vi "CalcCheckboxesFromTree.vi"(8 "error in (no error)":errorcluster, 11 "Tree Reference":refnum<vi>) -> (0 "error out":errorcluster, 1 "Element Status Conditions":T1(array[ring]), 2 "Element Values":enum8{"False", "True", "Mixed"}[](array[ring]))   [LabVIEW 2016, in "CS++MessageMakerMain.lvlib" / "CS++MessageMakerMain.lvclass"]
uses:
  CS++MessageMakerMain.lvclass
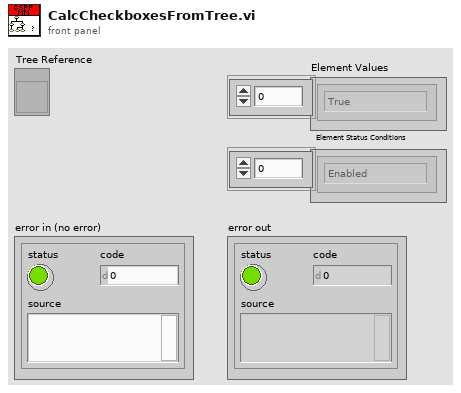
[diagram p1: front panel]
types:
  T1 = enum8{"Enabled", "Disabled", "Disabled and Grayed Out"}[]
  T2 = enum8{"Enabled", "Disabled", "Disabled and Grayed Out"}
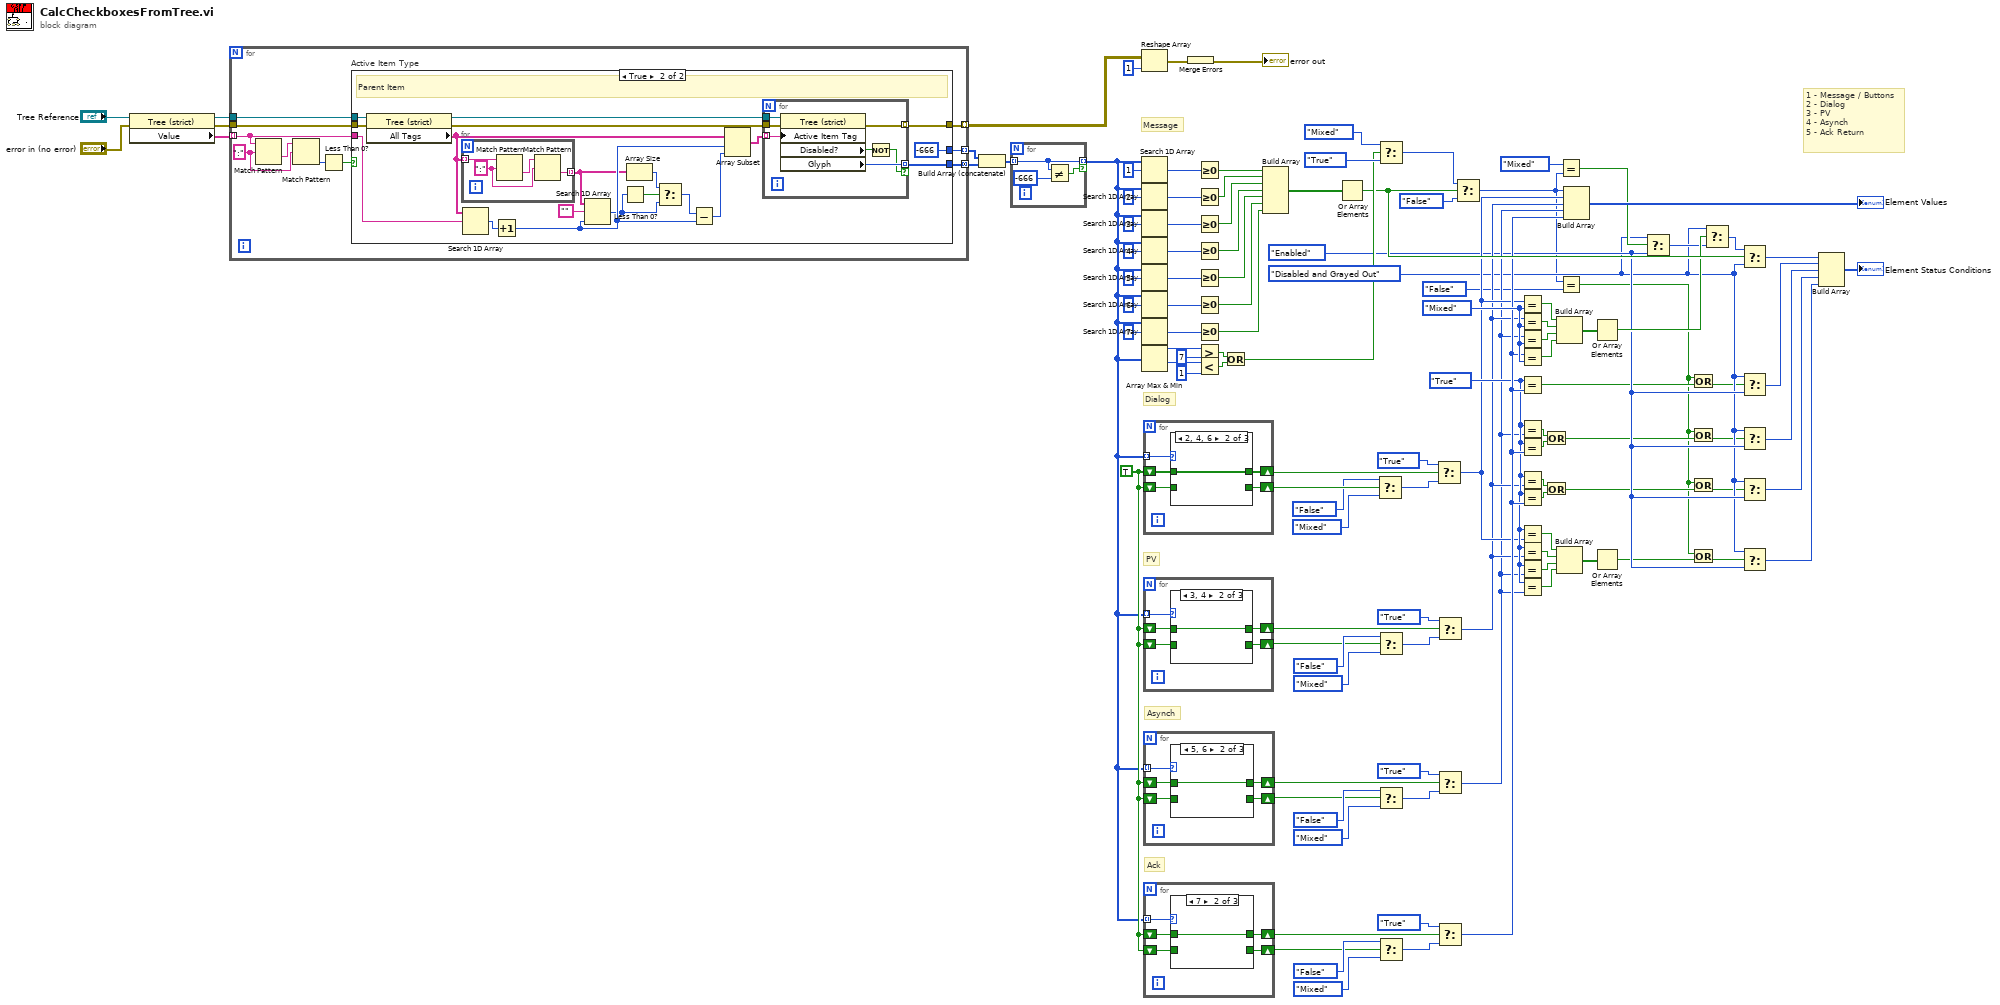
[diagram p0: block diagram]
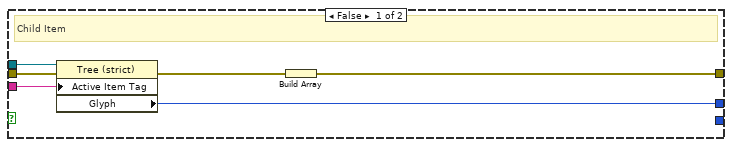
[diagram p2: hidden frame]
diagram:
  w24 = enum8{"False", "True", "Mixed"}."True" ("Element Value")
  w45 = enum8{"False", "True", "Mixed"}."Mixed" ("Element Value")
  w18 = T2."Enabled" ("Element Condition")
  w53 = TRUE
  w16 = T2."Disabled and Grayed Out" ("Element Condition")
  # "Message"
  # "Ack"
  # "Asynch"
  # "PV"
  # "Dialog"
  # "1 - Message / Buttons\n2 - Dialog\n3 - PV\n4 - Asynch\n5 - Ack Return"
  n1 = property class="Tree (strict)"(reference="Tree Reference", error in="error in (no error)") -> (reference out=w113:refnum<vi>, error out=w115:errorcluster, "Value"=w114:string[])
  n2 = for {
    tunnel: w114 -> [w123] mode=indexing
    tunnel: w113 -> [w121]
    tunnel: [w119] -> w15 mode=indexing
    tunnel: [w118] -> w14 mode=concatenating
    tunnel: w115 -> [w122]
    tunnel: [w120] -> w110 mode=indexing
    w126 = ":" ("regular expression")
    n3 = Match Pattern(string=w123, regular expression=w126) -> (after substring=w127:string)  [unwired: 1 in, 3 out]
    n4 = Match Pattern(string=w127, regular expression=w126) -> (offset past match=w125:i32)  [unwired: 1 in, 3 out]
    n5 = Less Than 0?(x=w125) -> (x < 0?=w124:bool)
    n6 = case "Active Item Type" shown="True" w124 {
      tunnel: w121 -> [w132 w152]
      tunnel: w123 -> [w129 w150]
      tunnel: w122 -> [w131 w151]
      tunnel: [w133 w141] -> w120
      tunnel: [_ w140] -> w118
      tunnel: [w128 -666 ("Glyph")] -> w119
      frame False {
        # "Child Item"
        n7 = property class="Tree (strict)"(reference=w132, error in=w131, "Active Item Tag"=w129) -> (error out=w130:errorcluster, "Glyph"=w128:i32)  [unwired: 1 out]
        n8 = Build Array(w130) -> (w133:errorcluster[])
      }
      frame True {
        # "Parent Item"
        n9 = property class="Tree (strict)"(reference=w152, error in=w151) -> (reference out=w144:refnum<vi>, error out=w143:errorcluster, "All Tags"=w147:string[])
        n10 = for {
          tunnel: w147 -> [w154] mode=indexing
          tunnel: [w153] -> w135 mode=indexing
          w155 = ":" ("regular expression")
          n11 = Match Pattern(string=w154, regular expression=w155) -> (after substring=w156:string)  [unwired: 1 in, 3 out]
          n12 = Match Pattern(string=w156, regular expression=w155) -> (after substring=w153:string)  [unwired: 1 in, 3 out]
        }
        n13 = Search 1D Array(1D array=w147, element=w150) -> (index of element=w149:i32)  [unwired: 1 in]
        n14 = Increment(x=w149) -> (x+1=w142:i32)
        n15 = Search 1D Array(1D array=w135, element="", start index (0)=w142) -> (index of element=w138:i32)
        n16 = Less Than 0?(x=w138) -> (x < 0?=w139:bool)
        n17 = Array Size(array=w135) -> (size(s)=w136:i32)
        n18 = Select(t=w136, s=w139, f=w138) -> (s? t:f=w137:i32)
        n19 = Subtract(x=w137, y=w142) -> (x-y=w146:i32)
        n20 = Array Subset(array=w147, index=w142, length=w146) -> (w145:string[])
        n21 = for {
          tunnel: w145 -> [w158] mode=indexing
          tunnel: w144 -> [w163]
          tunnel: w143 -> [w162]
          tunnel: [w160] -> w141 mode=indexing
          tunnel: [w159] -> w140 mode=indexing if=w157
          n22 = property class="Tree (strict)"(reference=w163, error in=w162, "Active Item Tag"=w158) -> (error out=w160:errorcluster, "Disabled?"=w161:bool, "Glyph"=w159:i32)  [unwired: 1 out]
          n23 = Not(x=w161) -> (.not. x?=w157:bool)
        }
      }
    }
  }
  n24 = Build Array (concatenate)(w15, w14) -> (w13:i32[])
  n25 = for {
    tunnel: w13 -> [w165] mode=indexing
    tunnel: [w165] -> w12 mode=indexing if=w164
    n26 = Not Equal?(x=w165, y=-666) -> (x != y?=w164:bool)
  }
  n27 = Reshape Array(w110, 1 ("dimension size")) -> (w111:errorcluster[])
  n28 = Search 1D Array(1D array=w12, element=1) -> (index of element=w101:i32)  [unwired: 1 in]
  n29 = Search 1D Array(1D array=w12, element=2) -> (index of element=w100:i32)  [unwired: 1 in]
  n30 = Search 1D Array(1D array=w12, element=3) -> (index of element=w99:i32)  [unwired: 1 in]
  n31 = Search 1D Array(1D array=w12, element=4) -> (index of element=w98:i32)  [unwired: 1 in]
  n32 = Search 1D Array(1D array=w12, element=5) -> (index of element=w97:i32)  [unwired: 1 in]
  n33 = Search 1D Array(1D array=w12, element=6) -> (index of element=w96:i32)  [unwired: 1 in]
  n34 = Search 1D Array(1D array=w12, element=7) -> (index of element=w95:i32)  [unwired: 1 in]
  n35 = Array Max & Min(array=w12) -> (max value=w81:i32, min value=w80:i32)  [unwired: 2 out]
  n36 = for {
    tunnel: w12 -> [w171] mode=indexing
    shift-right: [w169] -> w71
    shift-left: w53 -> [w170]
    shift-right: [w167] -> w68
    shift-left: w53 -> [w168]
    n37 = case shown="2, 4, 6" w171 {
      tunnel: w170 -> [w172 w174 _]
      tunnel: [w172 w174 _] -> w169
      tunnel: w168 -> [w173 _ w175]
      tunnel: [w173 _ w175] -> w167
      frame Default {
      }
      frame 2, 4, 6 {
      }
      frame 0, 1, 3, 5, 7 {
      }
    }
  }
  n38 = for {
    tunnel: w12 -> [w180] mode=indexing
    shift-right: [w178] -> w61
    shift-left: w53 -> [w179]
    shift-right: [w176] -> w60
    shift-left: w53 -> [w177]
    n39 = case shown="3, 4" w180 {
      tunnel: w179 -> [w181 w183 _]
      tunnel: [w181 w183 _] -> w178
      tunnel: w177 -> [w182 _ w184]
      tunnel: [w182 _ w184] -> w176
      frame Default {
      }
      frame 3, 4 {
      }
      frame 0..2, 5..7 {
      }
    }
  }
  n40 = for {
    tunnel: w12 -> [w189] mode=indexing
    shift-right: [w187] -> w55
    shift-left: w53 -> [w188]
    shift-right: [w185] -> w54
    shift-left: w53 -> [w186]
    n41 = case shown="5, 6" w189 {
      tunnel: w188 -> [w190 w192 _]
      tunnel: [w190 w192 _] -> w187
      tunnel: w186 -> [w191 _ w193]
      tunnel: [w191 _ w193] -> w185
      frame Default {
      }
      frame 5, 6 {
      }
      frame 0..4, 7 {
      }
    }
  }
  n42 = for {
    tunnel: w12 -> [w198] mode=indexing
    shift-right: [w196] -> w48
    shift-left: w53 -> [w197]
    shift-right: [w194] -> w47
    shift-left: w53 -> [w195]
    n43 = case shown="7" w198 {
      tunnel: w197 -> [w199 w201 _]
      tunnel: [w199 w201 _] -> w196
      tunnel: w195 -> [w200 _ w202]
      tunnel: [w200 _ w202] -> w194
      frame Default {
      }
      frame 7 {
      }
      frame 0..6 {
      }
    }
  }
  n44 = Merge Errors(w111) -> (→"error out":errorcluster)
  n45 = Greater Or Equal To 0?(x=w101) -> (x >= 0?=w88:bool)
  n46 = Greater Or Equal To 0?(x=w100) -> (x >= 0?=w87:bool)
  n47 = Greater Or Equal To 0?(x=w99) -> (x >= 0?=w86:bool)
  n48 = Greater Or Equal To 0?(x=w98) -> (x >= 0?=w85:bool)
  n49 = Greater Or Equal To 0?(x=w97) -> (x >= 0?=w84:bool)
  n50 = Greater Or Equal To 0?(x=w96) -> (x >= 0?=w83:bool)
  n51 = Greater Or Equal To 0?(x=w95) -> (x >= 0?=w82:bool)
  n52 = Greater?(x=w81, y=7) -> (0:w77:bool)
  n53 = Less?(x=w80, y=1) -> (x < y?=w76:bool)
  n54 = Or(x=w77, y=w76) -> (x .or. y?=w75:bool)
  n55 = Build Array(w88, w87, w86, w85, w84, w83, w82) -> (w72:bool[])
  n56 = Or Array Elements(Boolean array=w72) -> (logical OR=w73:bool)
  n57 = Select(t=enum8{"False", "True", "Mixed"}."False" ("Element Value"), s=w68, f=enum8{"False", "True", "Mixed"}."Mixed" ("Element Value")) -> (s? t:f=w69:enum8{"False", "True", "Mixed"})
  n58 = Select(t=enum8{"False", "True", "Mixed"}."Mixed" ("Element Value"), s=w75, f=enum8{"False", "True", "Mixed"}."True" ("Element Value")) -> (s? t:f=w93:enum8{"False", "True", "Mixed"})
  n59 = Select(t=enum8{"False", "True", "Mixed"}."False" ("Element Value"), s=w60, f=enum8{"False", "True", "Mixed"}."Mixed" ("Element Value")) -> (s? t:f=w63:enum8{"False", "True", "Mixed"})
  n60 = Select(t=enum8{"False", "True", "Mixed"}."False" ("Element Value"), s=w54, f=enum8{"False", "True", "Mixed"}."Mixed" ("Element Value")) -> (s? t:f=w58:enum8{"False", "True", "Mixed"})
  n61 = Select(t=enum8{"False", "True", "Mixed"}."False" ("Element Value"), s=w47, f=enum8{"False", "True", "Mixed"}."Mixed" ("Element Value")) -> (s? t:f=w50:enum8{"False", "True", "Mixed"})
  n62 = Select(t=enum8{"False", "True", "Mixed"}."True" ("Element Value"), s=w71, f=w69) -> (s? t:f=w23:enum8{"False", "True", "Mixed"})
  n63 = Select(t=enum8{"False", "True", "Mixed"}."True" ("Element Value"), s=w61, f=w63) -> (s? t:f=w22:enum8{"False", "True", "Mixed"})
  n64 = Select(t=enum8{"False", "True", "Mixed"}."True" ("Element Value"), s=w55, f=w58) -> (s? t:f=w21:enum8{"False", "True", "Mixed"})
  n65 = Select(t=enum8{"False", "True", "Mixed"}."True" ("Element Value"), s=w48, f=w50) -> (s? t:f=w31:enum8{"False", "True", "Mixed"})
  n66 = Select(t=w93, s=w73, f=enum8{"False", "True", "Mixed"}."False" ("Element Value")) -> (s? t:f=w10:enum8{"False", "True", "Mixed"})
  n67 = Equal?(x=w23, y=w45) -> (x = y?=w44:bool)
  n68 = Equal?(x=w22, y=w45) -> (x = y?=w43:bool)
  n69 = Equal?(x=w21, y=w45) -> (x = y?=w42:bool)
  n70 = Equal?(x=w31, y=w45) -> (x = y?=w41:bool)
  n71 = Equal?(x=w24, y=w31) -> (x = y?=w9:bool)
  n72 = Equal?(x=w24, y=w21) -> (x = y?=w36:bool)
  n73 = Equal?(x=w24, y=w31) -> (x = y?=w35:bool)
  n74 = Equal?(x=w24, y=w22) -> (x = y?=w32:bool)
  n75 = Equal?(x=w24, y=w31) -> (x = y?=w33:bool)
  n76 = Equal?(x=w24, y=w23) -> (x = y?=w25:bool)
  n77 = Equal?(x=w24, y=w22) -> (x = y?=w26:bool)
  n78 = Equal?(x=w24, y=w21) -> (x = y?=w27:bool)
  n79 = Equal?(x=w24, y=w21) -> (x = y?=w28:bool)
  n80 = Or(x=w36, y=w35) -> (x .or. y?=w7:bool)
  n81 = Or(x=w32, y=w33) -> (x .or. y?=w5:bool)
  n82 = Build Array(w44, w43, w42, w41) -> (w40:bool[])
  n83 = Build Array(w25, w26, w27, w28) -> (w29:bool[])
  n84 = Equal?(x=enum8{"False", "True", "Mixed"}."Mixed" ("Element Value"), y=w10) -> (x = y?=w19:bool)
  n85 = Equal?(x=w10, y=enum8{"False", "True", "Mixed"}."False" ("Element Value")) -> (x = y?=w3:bool)
  n86 = Build Array(w10, w23, w22, w21, w31) -> (→"Element Values":enum8{"False", "True", "Mixed"}[])
  n87 = Or Array Elements(Boolean array=w40) -> (logical OR=w39:bool)
  n88 = Or Array Elements(Boolean array=w29) -> (logical OR=w2:bool)
  n89 = Select(t=w16, s=w19, f=w18) -> (s? t:f=w17:T2)
  n90 = Or(x=w3, y=w9) -> (x .or. y?=w8:bool)
  n91 = Or(x=w3, y=w7) -> (x .or. y?=w6:bool)
  n92 = Or(x=w3, y=w5) -> (x .or. y?=w4:bool)
  n93 = Or(x=w3, y=w2) -> (x .or. y?=w1:bool)
  n94 = Select(t=w16, s=w39, f=w17) -> (s? t:f=w46:T2)
  n95 = Select(t=w46, s=w73, f=w16) -> (s? t:f=w74:T2)
  n96 = Select(t=w16, s=w8, f=w18) -> (s? t:f=w38:T2)
  n97 = Select(t=w16, s=w6, f=w18) -> (s? t:f=w37:T2)
  n98 = Select(t=w16, s=w4, f=w18) -> (s? t:f=w34:T2)
  n99 = Select(t=w16, s=w1, f=w18) -> (s? t:f=w30:T2)
  n100 = Build Array(w74, w38, w37, w34, w30) -> (→"Element Status Conditions":T1)
